vi "setupVersion_June30_TEMP.vi"() -> (6 "Instruments on/off":T1, 10 "error IO":errorcluster, 15 "OK":bool)   [LabVIEW 2014]
panel:
  in  "ok":bool
  in  "cancel":bool
  in  "Instruments connected":T2
  out "Keithley 2100 out":bool
  out "Pressure control 2":bool
  out "J-KEM2":bool
  out "Arduino2":bool
  out "Keithley 6431":bool
  out "Keithley 2421":bool
  out "SRS QCM 2":bool
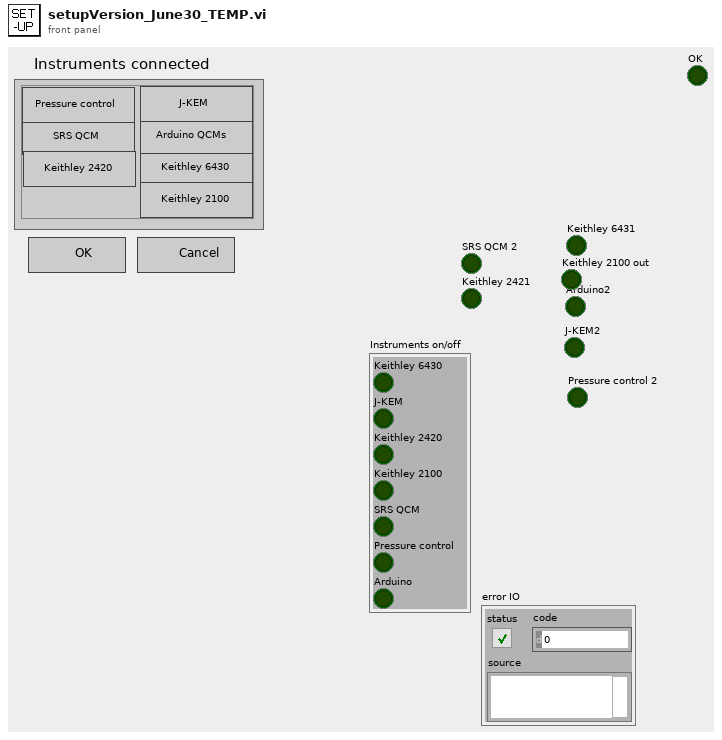
[diagram p1: front panel]
types:
  T1 = cluster{"Keithley 6430":bool, "J-KEM":bool, "Keithley 2420":bool, "Keithley 2100":bool, "SRS QCM":bool, "Pressure control":bool, "Arduino":bool}
  T2 = cluster{"SRS QCM":bool, "Keithley 2420":bool, "Keithley 6430":bool, "Keithley 2100":bool, "Arduino":bool, "J-KEM":bool, "Pressure control":bool}
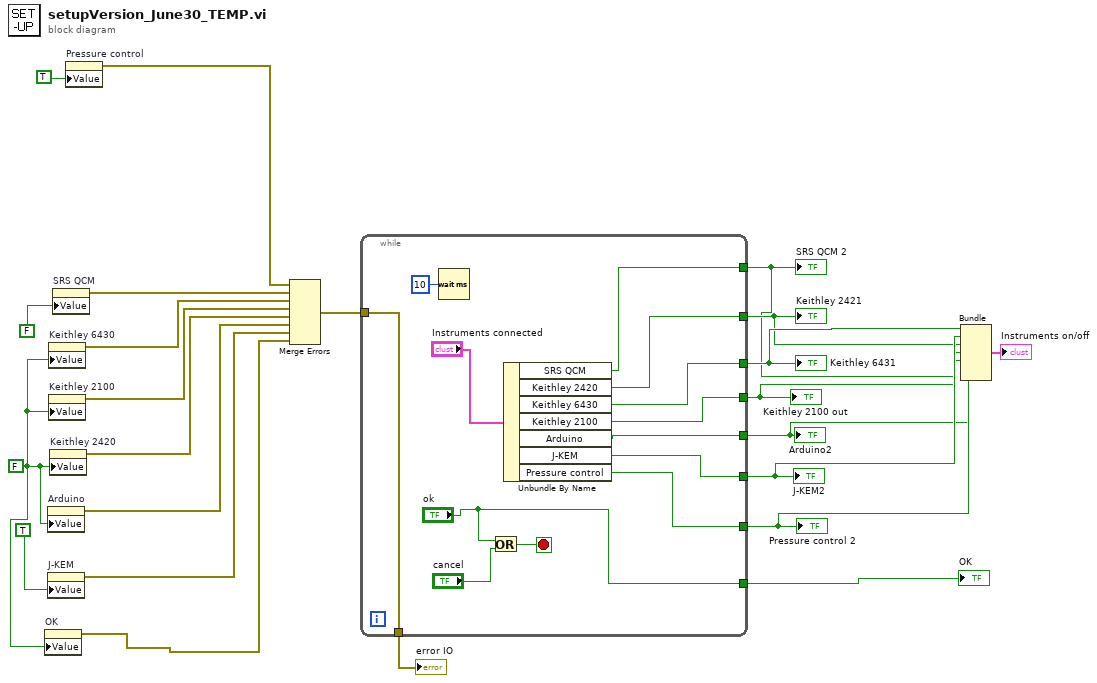
[diagram p0: block diagram]
diagram:
  w10 = FALSE ("Auto Stop")
  n1 = property on="OK" class="Bool (strict)"("Value"=w10) -> (error out=w9:errorcluster)  [unwired: 2 in, 1 out]
  n2 = property on="Arduino" class="Bool (strict)"("Value"=w10) -> (error out=w18:errorcluster)  [unwired: 2 in, 1 out]
  n3 = property on="J-KEM" class="Bool (strict)"("Value"=TRUE ("Auto Stop")) -> (error out=w17:errorcluster)  [unwired: 2 in, 1 out]
  n4 = property on="Keithley 6430" class="Bool (strict)"("Value"=w10) -> (error out=w20:errorcluster)  [unwired: 2 in, 1 out]
  n5 = property on="Keithley 2100" class="Bool (strict)"("Value"=w10) -> (error out=w12:errorcluster)  [unwired: 2 in, 1 out]
  n6 = property on="Keithley 2420" class="Bool (strict)"("Value"=w10) -> (error out=w22:errorcluster)  [unwired: 2 in, 1 out]
  n7 = property on="SRS QCM" class="Bool (strict)"("Value"=FALSE ("Auto Stop")) -> (error out=w19:errorcluster)  [unwired: 2 in, 1 out]
  n8 = property on="Pressure control" class="Bool (strict)"("Value"=TRUE ("Auto Stop")) -> (error out=w13:errorcluster)  [unwired: 2 in, 1 out]
  n9 = Merge Errors(w13, w19, w20, w12, w22, w18, w17, w9) -> (w23:errorcluster)
  n10 = while {
    tunnel: w23 -> [w35]
    tunnel: [w33] -> w4
    tunnel: [w32] -> w6
    tunnel: [w31] -> w8
    tunnel: [w29] -> w2
    tunnel: [w28] -> w7
    tunnel: [w27] -> w3
    tunnel: [w35] -> w14
    tunnel: [w30] -> w5
    tunnel: ["ok"] -> w11
    stop <- w25 stop-if-true
    n11 = Wait (ms)(milliseconds to wait=u32 10) -> ()  [unwired: 1 out]
    n12 = Or(x="ok", y="cancel") -> (x .or. y?=w25:bool)
    n13 = Unbundle By Name("Instruments connected") -> ("SRS QCM"=w33:bool, "Keithley 2420"=w32:bool, "Keithley 6430"=w31:bool, "Keithley 2100"=w30:bool, "Arduino"=w29:bool, "J-KEM"=w28:bool, "Pressure control"=w27:bool)
  }
  "SRS QCM 2" <- w4
  "Keithley 2421" <- w6
  "Keithley 6431" <- w8
  "Arduino2" <- w2
  "J-KEM2" <- w7
  "Pressure control 2" <- w3
  "error IO" <- w14
  "Keithley 2100 out" <- w5
  "OK" <- w11
  n14 = Bundle("Keithley 6430"=w8, "J-KEM"=w7, "Keithley 2420"=w6, "Keithley 2100"=w5, "SRS QCM"=w4, "Pressure control"=w3, "Arduino"=w2) -> (→"Instruments on/off":T1)  [unwired: 1 in]
